vi "Robot Global Data.vi"() -> ()   [LabVIEW 2014]
doc: "This global VI can contain as many global variables as you need. Place a control on the panel, give it a good name. To read or write to it from a VI, drag the icon to the diagram of that VI. You can also drag from the project. Click on the node to change which global you access. You shouldn't have multiple locations writing to a global or it will cause a race-condition."
uses:
  <vilib>/Rock Robotics/WPI/Camera/WPI_CameraImageSize.ctl
  <vilib>/Rock Robotics/WPI/DriverStation/WPI_DriverStationRobotMode2.ctl
panel:
  out "Manual":bool
  out "Gripper solenoid value":bool
  in  "Current Arm Case":dbl
  out "Release Can":bool
  in  "Wrist up position":dbl
  out "Gripper Enable":bool
  out "Can Sensor":bool
  out "Elevator up":bool
  out "Auton Array":dbl[][](array[numeric])
  in  "Arm Velocity":dbl
  in  "Wrist Offset":dbl=40.0
  in  "Desired Wrist Position":dbl
  in  "Current Wrist Position":dbl
  in  "Current Arm Position":dbl
  out "canGrabbed":bool
  out "Gripper Gripped":bool
  out "Grab Can":bool
  in  "Arm Sensor Offset":dbl=-120.0
  in  "Arm case":dbl
  in  "Desired Arm Position":dbl
  in  "Robot Mode":T1
  in  "image size":T2=enum."320x240"
  in  "Enable Vision":bool
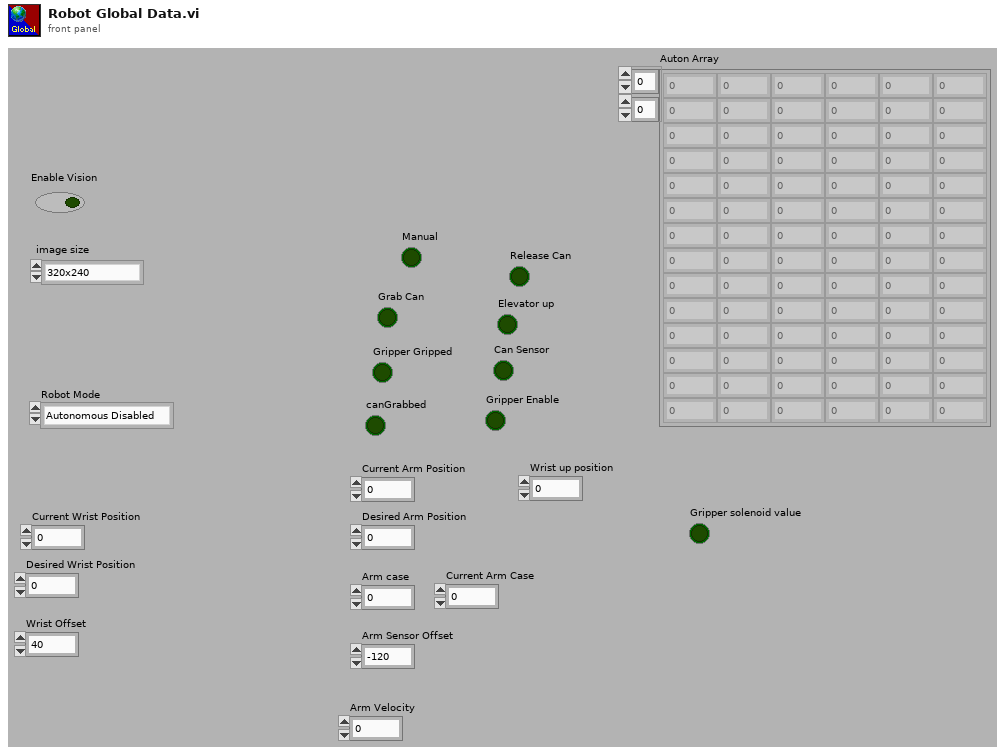
[diagram p1: front panel]
types:
  T1 = typedef "WPI_DriverStationRobotMode2.ctl" = enum16{"Autonomous Disabled", "Autonomous Enabled", "Teleop Disabled", "Teleop Enabled", "Disconnected", "Finish", "Test Disabled", "Test Enabled", "Emergency Stopped"}
  T2 = typedef "WPI_CameraImageSize.ctl" = enum16{"640x480", "320x240", "160x120", "Custom"}
diagram:
